vi "average projected images.vi"(7 "reset?":bool, 9 "num frames":u8=10 min=1, 10 "averaging mode":enum16{"exponential", "linear"}(ring), 11 "projections":T2) -> (1 "in loop reset":bool, 2 "reset":bool, 3 "averaged projections":T1)   [LabVIEW 2010]
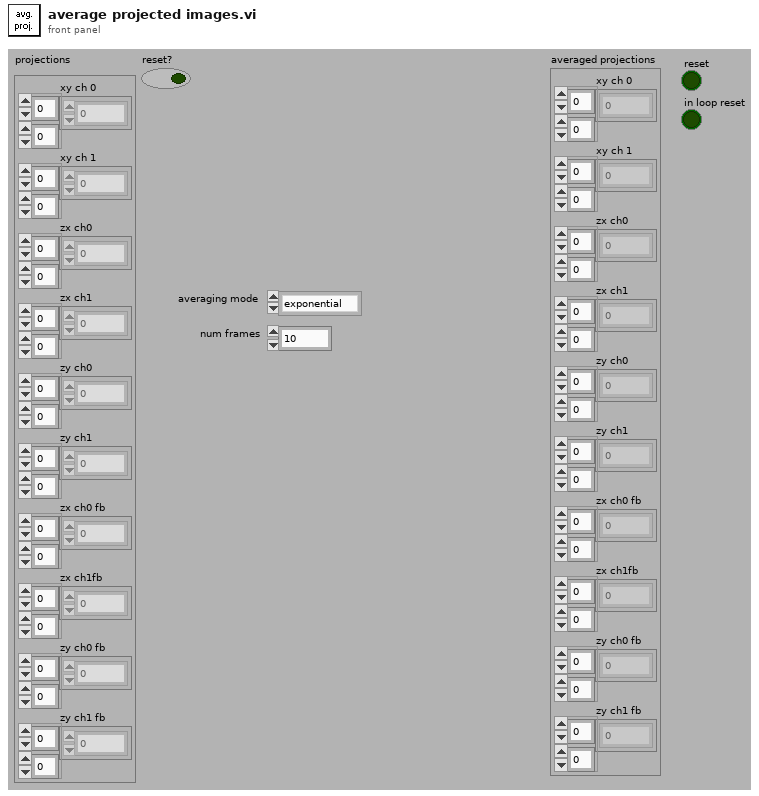
[diagram p1: front panel]
types:
  T1 = cluster{"xy ch 0":u16[][], "xy ch 1":u16[][], "zx ch0":u16[][], "zx ch1":u16[][], "zy ch0":u16[][], "zy ch1":u16[][], "zx ch0 fb":u16[][], "zx ch1fb":u16[][], "zy ch0 fb":u16[][], "zy ch1 fb":u16[][]}
  T2 = cluster{"xy ch 0":dbl[][], "xy ch 1":dbl[][], "zx ch0":dbl[][], "zx ch1":dbl[][], "zy ch0":dbl[][], "zy ch1":dbl[][], "zx ch0 fb":dbl[][], "zx ch1fb":dbl[][], "zy ch0 fb":dbl[][], "zy ch1 fb":dbl[][]}
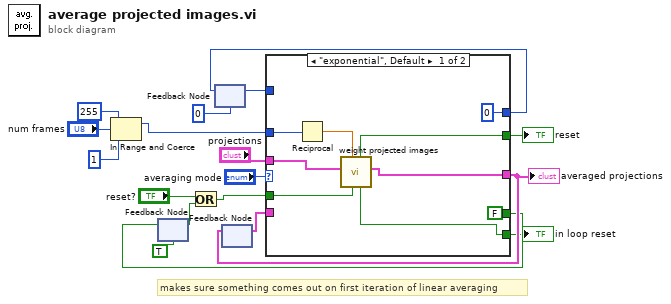
[diagram p0: block diagram]
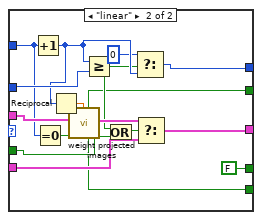
[diagram p2: hidden frame]
diagram:
  # "makes sure something comes out on first iteration of linear averaging"
  n1 = In Range and Coerce(upper limit=u8 255, x="num frames", lower limit=u8 1) -> (coerced(x)=w7:u8)  [unwired: 1 out]
  n2 = feedback #1(TRUE) -> (w9:bool)
  n3 = Or(x="reset?", y=w9) -> (x .or. y?=w4:bool)
  n4 = feedback #2(0) -> (w14:i32)
  n5 = feedback #3() -> (w11:T1)  [unwired: 1 in]
  n6 = case shown="\"exponential\", Default" "averaging mode" {
    tunnel: "projections" -> [w27 w43]
    tunnel: w7 -> [w26 w44]
    tunnel: w14 -> [_ w32]
    tunnel: [0 ("t") w39] -> w13
    tunnel: [w24 w37] -> w12
    tunnel: w11 -> [_ w36]
    tunnel: w4 -> [w21 w31]
    tunnel: [FALSE FALSE] -> w8
    tunnel: [w20 w29] -> w2
    tunnel: [w19 w28] -> w1
    frame "exponential", Default {
      n7 = Reciprocal(x=w26) -> (1/x=w25:dbl)
      n8 = call "weight projected images.vi"("reset?"=w21, "weight"=w25, "projections"=w27) -> ("projections out"=w24:T1, "in loop reset"=w19:bool, "reset"=w20:bool)  [unwired: 6 in]
    }
    frame "linear" {
      n9 = Increment(x=w32) -> (x+1=w41:i32)
      n10 = Equal To 0?(x=w32) -> (x = 0?=w30:bool)
      n11 = Reciprocal(x=w41) -> (1/x=w42:dbl)
      n12 = call "weight projected images.vi"("reset?"=w30, "weight"=w42, "projections"=w43) -> ("projections out"=w38:T1, "in loop reset"=w28:bool, "reset"=w29:bool)  [unwired: 6 in]
      n13 = Greater Or Equal?(x=w41, y=w44) -> (x >= y?=w34:bool)
      n14 = Or(x=w34, y=w31) -> (x .or. y?=w35:bool)
      n15 = Select(t=0, s=w34, f=w41) -> (s? t:f=w39:i32)
      n16 = Select(t=w38, s=w35, f=w36) -> (s? t:f=w37:T1)
    }
  }
  "averaged projections" <- w12
  "reset" <- w2
  "in loop reset" <- w1
  n17 = feedback-in #1(w8) -> ()
  n18 = feedback-in #2(w13) -> ()
  n19 = feedback-in #3(w12) -> ()
